vi "Tmp_M open msg.vi"(8 "error in (no error)":errorcluster, 9 "timeout ms (1000)":i32=1000, 10 "Connected":bool, 11 "Queue in":T2) -> (0 "error out":errorcluster, 1 "timed out?":bool, 2 "Data":variant, 3 "Command":T1, 5 "Unread":i32)   [LabVIEW 2021, in "Temperature monitor.lvlib"]
uses:
  Temperature monitor.lvlib
  Messenger service/MessengerLib.lvlib
  Typedefs/Tmp_M commands.ctl
  ctl/MSG to Tmp_M.ctl
  Magnet module.lvlib
  Messenger service/Data types/Mailbox address.ctl
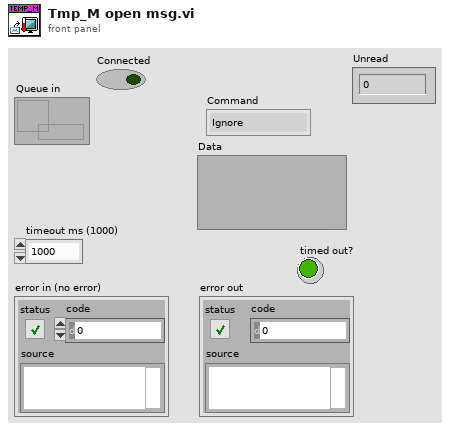
[diagram p1: front panel]
types:
  T1 = typedef "Temperature monitor.lvlib/Tmp_M commands.ctl" = enum16{"Ignore", "Connect", "Set timeout", "Update", "Disconnect"}
  T2 = typedef "MessengerLib.lvlib/Mailbox address.ctl" = refnum<queue>
  T3 = typedef "Magnet module.lvlib/MSG to Tmp_M.ctl" = cluster{"Command":T1, "Data":variant}
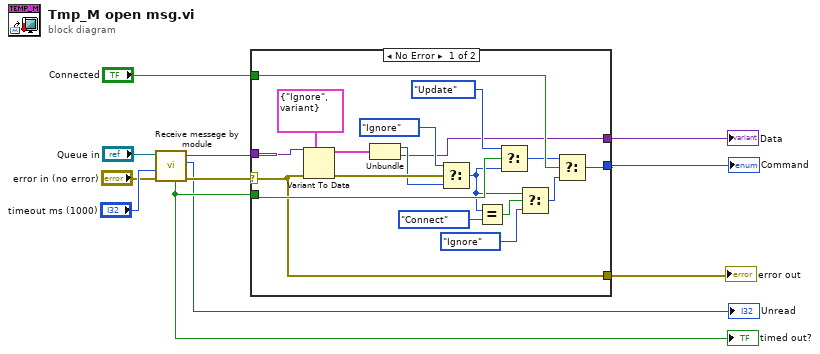
[diagram p0: block diagram]
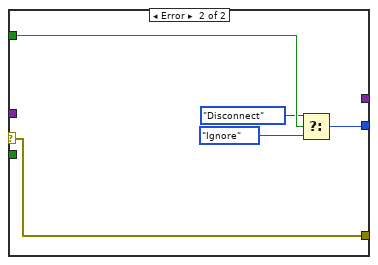
[diagram p2: hidden frame]
diagram:
  n1 = call "Receive messege by module.vi"("error in (no error)"="error in (no error)", "timeout in ms (-1)"="timeout ms (1000)", "Module mailbox"="Queue in") -> ("error out"=w6:errorcluster, "Unread"=→"Unread":i32, "Data"=w7:variant, "timed out?"=w5:bool)  [unwired: 4 in, 1 out]
  "timed out?" <- w5
  n2 = case shown="No Error" w6 {
    selector: w6 -> [w16 w34]
    tunnel: w5 -> [w28 _]
    tunnel: [w16 w34] -> w3
    tunnel: "Connected" -> [w29 w31]
    tunnel: w7 -> [w21 _]
    tunnel: [w17 w32] -> w2
    tunnel: [w12 _] -> w4
    frame No Error {
      n3 = Variant To Data(error in=w16, type=T3 {"Command"=enum."Ignore", "Data"=variant}, Variant=w21) -> (data=w18:T3, error out=w19:errorcluster)
      n4 = Unbundle(w18) -> ("Command"=w14:T1, "Data"=w12:variant)
      n5 = Select(t=Tmp_M_commands."Ignore" ("Command"), s=w19, f=w14) -> (s? t:f=w13:T1)
      n6 = Equal?(x=w13, y=Tmp_M_commands."Connect" ("Command")) -> (x = y?=w24:bool)
      n7 = Select(t=Tmp_M_commands."Update" ("Command"), s=w28, f=w13) -> (s? t:f=w26:T1)
      n8 = Select(t=w13, s=w24, f=Tmp_M_commands."Ignore" ("Command")) -> (s? t:f=w23:T1)
      n9 = Select(t=w26, s=w29, f=w23) -> (s? t:f=w17:T1)
    }
    frame Error {
      n10 = Select(t=Tmp_M_commands."Disconnect", s=w31, f=Tmp_M_commands."Ignore" ("Command")) -> (s? t:f=w32:T1)
    }
  }
  "error out" <- w3
  "Data" <- w4
  "Command" <- w2
